vi "Nav6 Example.vi"() -> ()   [LabVIEW 2014]
uses:
  Nav6Library/CalibrationState.ctl
  Nav6Library/Nav6.lvlib
panel:
  out "Open Succesfull":bool
  out "Accelerometer Full Scale Range":u32
  out "Gyroscope Full Scale Range":u32
  out "CalibrationState":T1
  out "IsConnected":bool
  out "Byte Count":u32
  out "Update Count":i32
  out "Compass Heading":dbl
  out "Roll":dbl
  out "Pitch":dbl
  in  "Zero Yaw":bool
  out "Yaw":dbl
  in  "stop":bool
  in  "UpdateRate (Hz)":u8=100
  # "Outputs from Open"
  # "Set this input\nbefore running"
  # "Outputs"
  # "This can be set \nwhile running"
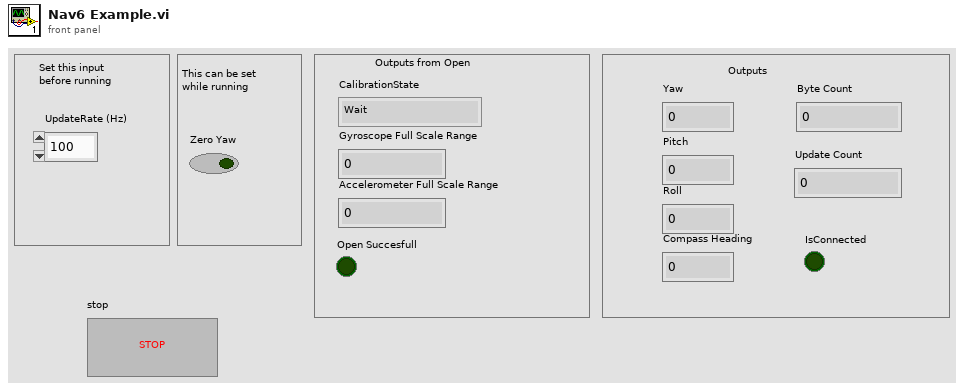
[diagram p1: front panel]
types:
  T1 = typedef "Nav6.lvlib/CalibrationState.ctl" = enum16{"Wait", "Accumulate", "Complete"}
  T2 = typedef "WPI_SerialPortRef.ctl" = cluster{"DevStatus":errorcluster, "Serial Port Name":refnum<visa-resource-name>}
  T3 = typedef "Nav6.lvlib/Nav6DevRef.ctl" = cluster{"SerialPortRef":T2, "UpdateRate":u8, "Error":errorcluster, "Nav6Mode":T4}
  T4 = typedef "Nav6.lvlib/Nav6Mode.ctl" = enum16{"YPR", "Gyro", "Quaternion"}
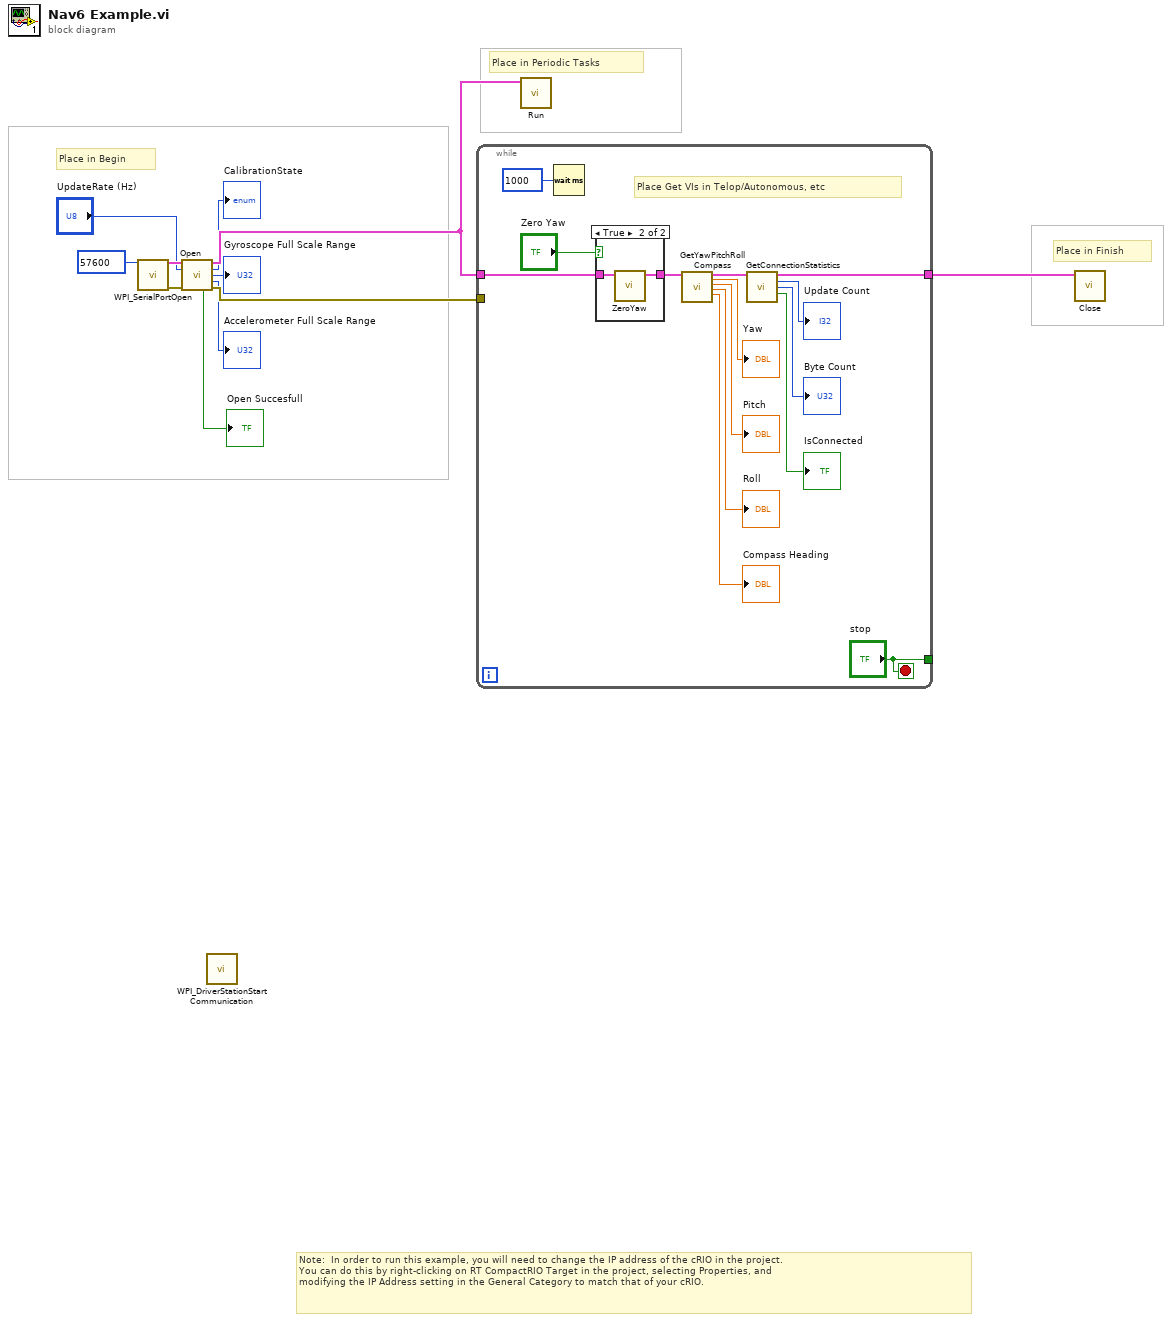
[diagram p0: block diagram]
diagram:
  # "Place in Finish"
  # "Place in Periodic Tasks"
  # "Place in Begin"
  # "Note:  In order to run this example, you will need to change the IP address of the cRIO in the project.  \nYou can do this by right-clicking on RT CompactRIO Target in the project, selecting Properties, and \nmodifying the IP Address setting in the General Category to match that of your cRIO."
  n1 = call <vilib>:"WPI_SerialPortOpen.vi"("Baud Rate"=u32 57600) -> ("SerialPortRef"=w11:T2, "error out"=w7:errorcluster)  [unwired: 13 in]
  n2 = call "Open.vi"("SerialPortRef"=w11, "UpdateRate (100Hz)"="UpdateRate (Hz)", "error in (no error)"=w7) -> ("Nav6DevRef"=w8:T3, "CalibrationState"=→"CalibrationState":T1, "Gyroscope Full Scale Range (deg/sec)"=→"Gyroscope Full Scale Range":u32, "Accelerometer Full Scale Range (g)"=→"Accelerometer Full Scale Range":u32, "Open Succesfull"=→"Open Succesfull":bool, "error out"=w5:errorcluster)  [unwired: 6 in, 1 out]
  n3 = call <vilib>:"WPI_DriverStationStart Communication.vi"() -> ()  [unwired: 12 in]
  n4 = while {
    tunnel: w8 -> [w18]
    tunnel: ["stop"] -> _
    tunnel: [w16] -> w6
    tunnel: w5 -> [_]
    stop <- "stop" stop-if-true
    # "Place Get VIs in Telop/Autonomous, etc"
    n5 = Wait (ms)(milliseconds to wait=u32 1000) -> ()  [unwired: 1 out]
    n6 = case shown="True" "Zero Yaw" {
      tunnel: [w26 w28] -> w19
      tunnel: w18 -> [w26 w27]
      frame False {
      }
      frame True {
        n7 = call "ZeroYaw.vi"("Nav6DevRef"=w27) -> ("Nav6DevRef Out"=w28:T3)  [unwired: 9 in, 1 out]
      }
    }
    n8 = call "GetYawPitchRollCompass.vi"("Nav6DevRef"=w19) -> ("Nav6DevRef Out"=w17:T3, "Yaw"=→"Yaw":dbl, "Pitch"=→"Pitch":dbl, "Roll"=→"Roll":dbl, "Compass Heading"=→"Compass Heading":dbl)  [unwired: 12 in, 2 out]
    n9 = call "GetConnectionStatistics.vi"("Nav6DevRef"=w17) -> ("Nav6DevRef Out"=w16:T3, "Update Count"=→"Update Count":i32, "Byte Count"=→"Byte Count":u32, "IsConnected"=→"IsConnected":bool)  [unwired: 10 in, 1 out]
  }
  n10 = call "Run.vi"("Nav6DevRef"=w8) -> ()  [unwired: 11 in]
  n11 = call "Close.vi"("Nav6DevRef"=w6) -> ()  [unwired: 10 in, 1 out]
